vi "Close.vi"(8 "error in (no error)":errorcluster, 11 "MODBUS in":refnum<class "PL Modbus Client.lvclass">) -> (0 "error out":errorcluster)   [LabVIEW 2015, in "PL Modbus Client.lvclass"]
doc: "Closes connection to Modbus server."
uses:
  PL Modbus Client.lvclass
  PL Modbus Client.lvclass/PL Modbus Client.ctl
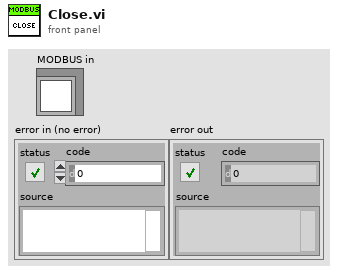
[diagram p1: front panel]
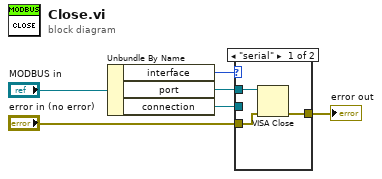
[diagram p0: block diagram]
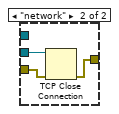
[diagram p2: hidden frame]
diagram:
  n1 = Unbundle By Name("MODBUS in") -> ("interface"=w5:enum16{"serial", "network"}, "port"=w3:refnum<visa-resource-name>, "connection"=w4:refnum<k5>)
  n2 = case shown="\"serial\"" w5 {
    tunnel: w4 -> [_ w12]
    tunnel: w3 -> [w9 _]
    tunnel: [w8 w11] -> w2
    tunnel: "error in (no error)" -> [w7 w10]
    frame "serial" {
      n3 = VISA Close(VISA resource name=w9, error in (no error)=w7) -> (error out=w8:errorcluster)
    }
    frame "network" {
      n4 = TCP Close Connection(connection ID=w12, error in (no error)=w10) -> (error out=w11:errorcluster)  [unwired: 1 in, 1 out]
    }
  }
  "error out" <- w2
